vi "SetTo0.vi"(10 "Longueur d'onde":dbl) -> (2 "Température 0":dbl)   [LabVIEW 2018]
uses:
  <vilib>/DAQmx/write.llb/DAQmx Write (Digital 1D Bool NChan 1Samp 1Line).vi
  <vilib>/DAQmx/read.llb/DAQmx Read (Analog 1D Wfm NChan NSamp).vi
  <vilib>/Analysis/baseanly.llb/Mean (DBL).vi
  <vilib>/DAQmx/create/channels.llb/DAQmx Create Channel (DO-Digital Output).vi
  <vilib>/DAQmx/miscellaneous.llb/DAQmx Fill In Error Info.vi
  <vilib>/DAQmx/create/channels.llb/DAQmx Create Channel (AI-Voltage-Basic).vi
  <vilib>/DAQmx/configure/timing.llb/DAQmx Timing (Sample Clock).vi
  <vilib>/Analysis/NI_AALBase.lvlib
  <resource>/objmgr/daqmx.rc
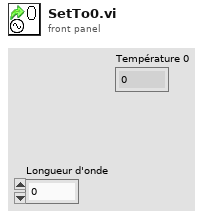
[diagram p1: front panel]
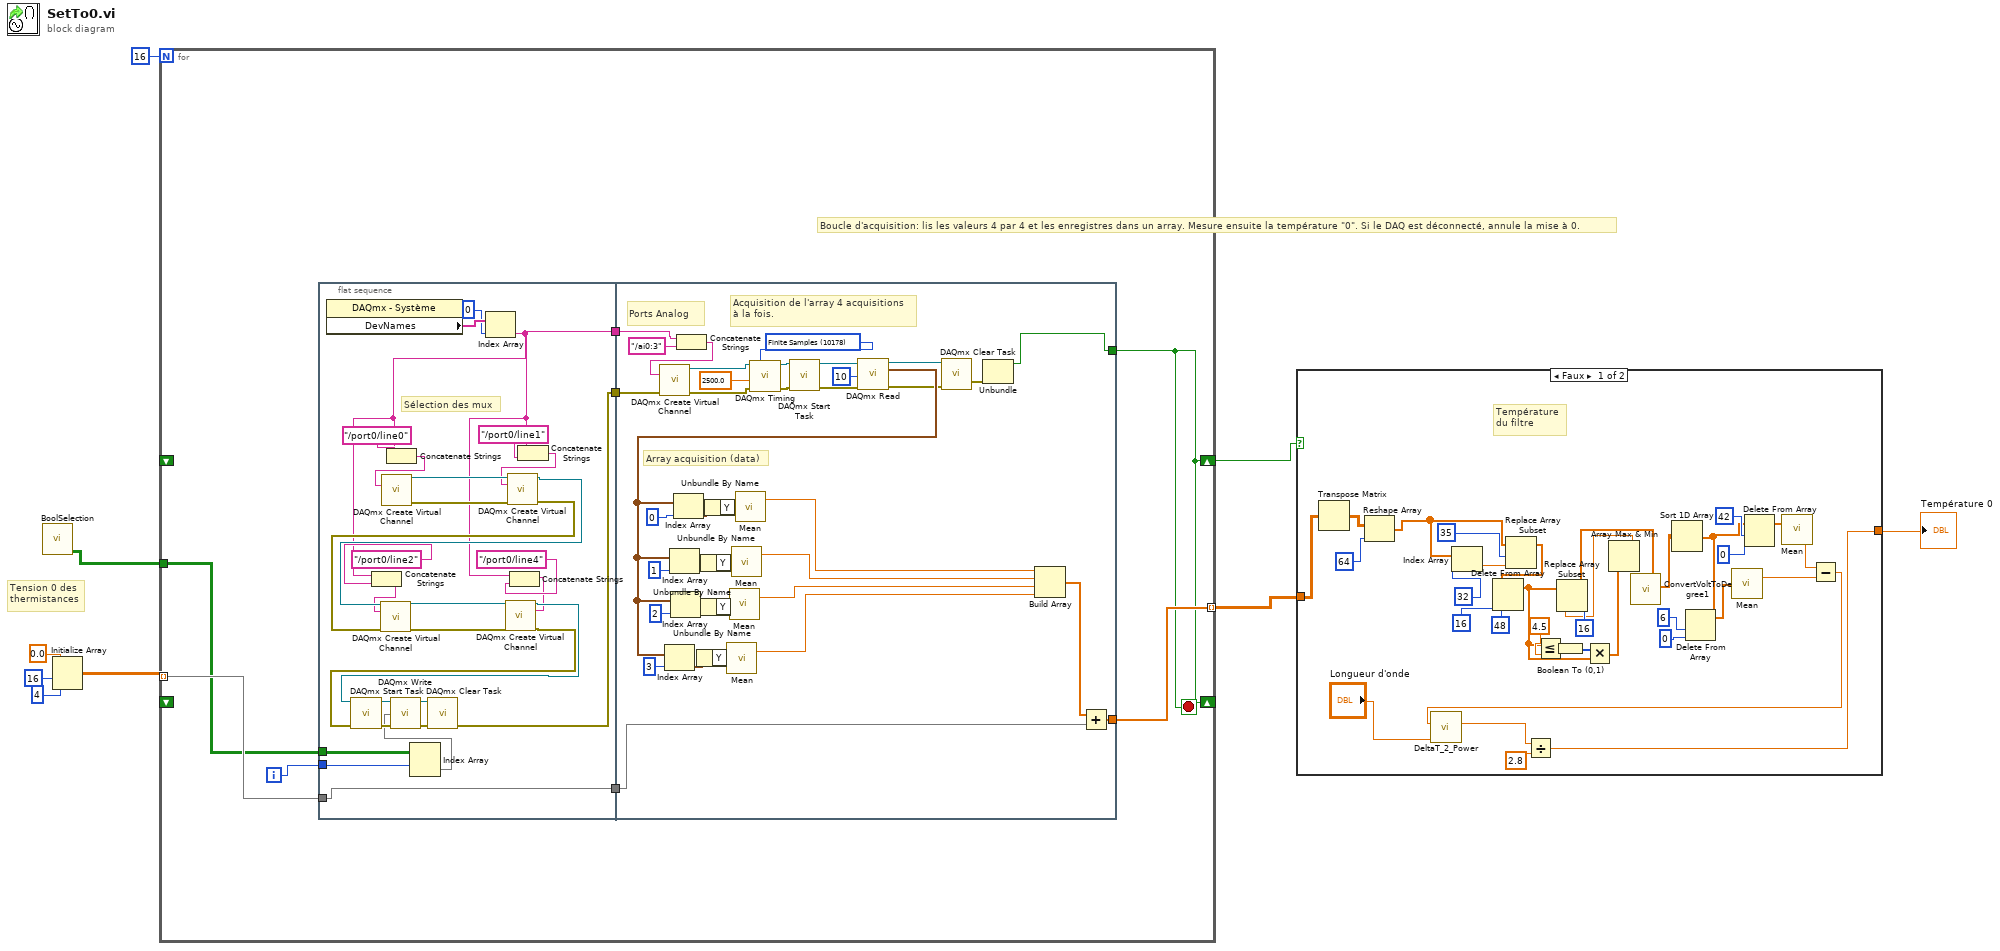
[diagram p0: block diagram]
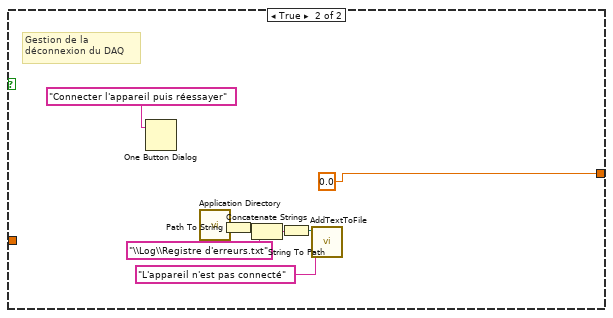
[diagram p2: hidden frame]
diagram:
  # "Tension 0 des \nthermistances"
  # "Boucle d'acquisition: lis les valeurs 4 par 4 et les enregistres dans un array. Mesure ensuite la température \"0\". Si le DAQ est déconnecté, annule la mise à 0."
  n1 = call "BoolSelection.vi"() -> ("BoolSelection"=w2:bool[][])  [unwired: 11 in]
  n2 = Initialize Array(0.0 ("element"), 16 ("dimension size"), 4 ("dimension size")) -> (w3:dbl[][])
  n3 = for {
    N: 16 -> [_]
    tunnel: w2 -> [w12]
    tunnel: w3 -> [w17] mode=indexing
    tunnel: [w11] -> w8 mode=indexing
    shift-right: [w10] -> _
    shift-left: _ -> [_]
    shift-right: [w10] -> w9
    shift-left: _ -> [_]
    i -> [w13]
    stop <- w10 stop-if-true
    n4 = flat-sequence {
      tunnel: w13 -> [w31]
      tunnel: [w42] -> w16
      tunnel: w12 -> [w30]
      tunnel: [w18] -> w15
      tunnel: [w19] -> w14
      tunnel: w17 -> [w18]
      tunnel: w16 -> [w74]
      tunnel: w15 -> [w54]
      tunnel: [w56] -> w11
      tunnel: w14 -> [w51]
      tunnel: [w46] -> w10
      frame #0 {
        # "Sélection des mux"
        n5 = property class="DAQmx - Système"() -> ("DevNames"=w29:tag[])  [unwired: 2 in, 2 out]
        n6 = Index Array(array=w30, index (row)=w31) -> (element=w43:bool[])  [unwired: 1 in]
        n7 = Index Array(array=w29, index=0) -> (element=w19:tag)
        n8 = Concatenate Strings(w19, "/port0/line2" ("string")) -> (w22:string)
        n9 = Concatenate Strings(w19, "/port0/line0" ("string")) -> (w27:string)
        n10 = call-poly <vilib>:"DAQmx Create Virtual Channel.vi"("lines"=w27) -> ("task out"=w38:refnum<k21>, "error out"=w39:errorcluster)  [unwired: 13 in]
        n11 = Concatenate Strings(w19, "/port0/line4" ("string")) -> (w20:string)
        n12 = Concatenate Strings(w19, "/port0/line1" ("string")) -> (w24:string)
        n13 = call-poly <vilib>:"DAQmx Create Virtual Channel.vi"("task in"=w38, "lines"=w24, "error in"=w39) -> ("task out"=w37:refnum<k21>, "error out"=w36:errorcluster)  [unwired: 11 in]
        n14 = call-poly <vilib>:"DAQmx Create Virtual Channel.vi"("task in"=w37, "lines"=w22, "error in"=w36) -> ("task out"=w34:refnum<k21>, "error out"=w35:errorcluster)  [unwired: 11 in]
        n15 = call-poly <vilib>:"DAQmx Create Virtual Channel.vi"("task in"=w34, "lines"=w20, "error in"=w35) -> ("task out"=w33:refnum<k21>, "error out"=w32:errorcluster)  [unwired: 11 in]
        n16 = call <vilib>:"DAQmx Start Task.vi"("task/channels in"=w33, "error in"=w32) -> ("task out"=w44:refnum<k21>, "error out"=w45:errorcluster)  [unwired: 12 in]
        n17 = call-poly <vilib>:"DAQmx Write.vi"("task/channels in"=w44, "data"=w43, "error in"=w45) -> ("task out"=w41:refnum<k21>, "error out"=w40:errorcluster)  [unwired: 10 in, 1 out]
        n18 = call <vilib>:"DAQmx Clear Task.vi"("task in"=w41, "error in"=w40) -> ("error out"=w42:errorcluster)  [unwired: 13 in]
      }
      frame #1 {
        w76 = 10178 items=["Finite Samples"=10178, "Continuous Samples"=10123, "Hardware Timed Single Point"=12522] ("sample mode")
        # "Ports Analog"
        # "Array acquisition (data)"
        # "Acquisition de l'array 4 acquisitions\nà la fois."
        n19 = Concatenate Strings(w51, "/ai0:3" ("string")) -> (w52:string)
        n20 = call-poly <vilib>:"DAQmx Create Virtual Channel.vi"("physical channels"=w52, "error in"=w74) -> ("task out"=w81:refnum<k21>, "error out"=w80:errorcluster)  [unwired: 12 in]
        n21 = call-poly <vilib>:"DAQmx Timing.vi"("task/channels in"=w81, "sample mode"=w76, "rate"=2500.0, "error in"=w80) -> ("task out"=w77:refnum<k21>, "error out"=w78:errorcluster)  [unwired: 10 in]
        n22 = call <vilib>:"DAQmx Start Task.vi"("task/channels in"=w77, "error in"=w78) -> ("task out"=w79:refnum<k21>, "error out"=w82:errorcluster)  [unwired: 12 in]
        n23 = call-poly <vilib>:"DAQmx Read.vi"("task/channels in"=w79, "number of samples per channel"=10, "error in"=w82) -> ("task out"=w58:refnum<k21>, "data"=w67:waveform(dbl)[], "error out"=w57:errorcluster)  [unwired: 10 in]
        n24 = Index Array(array=w67, index=3) -> (element=w63:waveform(dbl))
        n25 = Index Array(array=w67, index=1) -> (element=w65:waveform(dbl))
        n26 = Index Array(array=w67, index=2) -> (element=w64:waveform(dbl))
        n27 = Index Array(array=w67, index=0) -> (element=w66:waveform(dbl))
        n28 = Unbundle By Name(w63) -> ("Y"=w59:dbl[])
        n29 = Unbundle By Name(w65) -> ("Y"=w61:dbl[])
        n30 = Unbundle By Name(w64) -> ("Y"=w60:dbl[])
        n31 = Unbundle By Name(w66) -> ("Y"=w62:dbl[])
        n32 = call-poly <vilib>:"Mean.vi"("X"=w59) -> ("mean"=w47:dbl)  [unwired: 1 out]
        n33 = call-poly <vilib>:"Mean.vi"("X"=w60) -> ("mean"=w48:dbl)  [unwired: 1 out]
        n34 = call-poly <vilib>:"Mean.vi"("X"=w61) -> ("mean"=w49:dbl)  [unwired: 1 out]
        n35 = call-poly <vilib>:"Mean.vi"("X"=w62) -> ("mean"=w50:dbl)  [unwired: 1 out]
        n36 = call <vilib>:"DAQmx Clear Task.vi"("task in"=w58, "error in"=w57) -> ("error out"=w72:errorcluster)  [unwired: 13 in]
        n37 = Unbundle(w72) -> ("status"=w46:bool)  [unwired: 2 out]
        n38 = Build Array(w50, w49, w48, w47) -> (w55:dbl[])
        n39 = Add(x=w55, y=w54) -> (x+y=w56:dbl[])
      }
    }
  }
  n40 = case shown="Faux" w9 {
    tunnel: w8 -> [w114 _]
    tunnel: [w84 0.0] -> w1
    frame False {
      # "Température \ndu filtre"
      n41 = Transpose Matrix(1:w114) -> (0:w115:dbl[][])
      n42 = Reshape Array(w115, 64 ("dimension size")) -> (w83:dbl[])
      n43 = Index Array(array=w83, index=32) -> (element=w92:dbl)
      n44 = Replace Array Subset(array=w83, new element=w92, index=35) -> (w103:dbl[])
      n45 = Delete From Array(array=w103, length=16, index=48) -> (array with subset deleted=w102:dbl[])  [unwired: 1 out]
      n46 = Less Or Equal?(x=w102, y=4.5) -> (x <= y?=w107:bool[])
      n47 = Boolean To (0,1)(Boolean=w107) -> (0, 1=w106:i16[])
      n48 = Multiply(x=w106, y=w102) -> (x*y=w105:dbl[])
      n49 = Array Max & Min(array=w105) -> (max value=w101:dbl)  [unwired: 3 out]
      n50 = Replace Array Subset(array=w102, new element=w101, index=16) -> (w93:dbl[])
      n51 = call "ConvertVoltToDegree1.vi"("Tension"=w93) -> ("Température"=w91:dbl[])  [unwired: 10 in]
      n52 = Sort 1D Array(array=w91) -> (sorted array=w90:dbl[])
      n53 = Delete From Array(array=w90, length=6, index=0) -> (array with subset deleted=w95:dbl[])  [unwired: 1 out]
      n54 = call-poly <vilib>:"Mean.vi"("X"=w95) -> ("mean"=w89:dbl)  [unwired: 1 out]
      n55 = Delete From Array(array=w90, length=42, index=0) -> (array with subset deleted=w98:dbl[])  [unwired: 1 out]
      n56 = call-poly <vilib>:"Mean.vi"("X"=w98) -> ("mean"=w94:dbl)  [unwired: 1 out]
      n57 = Subtract(x=w94, y=w89) -> (x-y=w88:dbl)
      n58 = call "DeltaT_2_Power.vi"("Longueur d'onde"="Longueur d'onde", "Delta T"=w88) -> ("Power"=w85:dbl)  [unwired: 9 in]
      n59 = Divide(x=w85, y=2.8) -> (x/y=w84:dbl)
    }
    frame True {
      # "Gestion de la \ndéconnexion du DAQ"
      n60 = One Button Dialog(message="Connecter l'appareil puis réessayer") -> ()  [unwired: 1 in, 1 out]
      n61 = call <vilib>:"Application Directory.vi"() -> ("Application Directory"=w120:path)
      n62 = Path To String(path=w120) -> (string=w121:string)
      n63 = Concatenate Strings(w121, "\\Log\\Registre d'erreurs.txt") -> (w122:string)
      n64 = String To Path(string=w122) -> (path=w118:path)
      n65 = call "AddTextToFile.vi"("Ajouter du texte"="L'appareil n'est pas connecté", "Fichier"=w118) -> ()  [unwired: 10 in]
    }
  }
  "Température 0" <- w1
